vi "sum line into array.vi"(9 "insert location":i32, 10 "array to sum in":u32[](array[numeric]), 11 "array":u32[](array[numeric])) -> (3 "array out":u32[](array[numeric]))   [LabVIEW 2010]
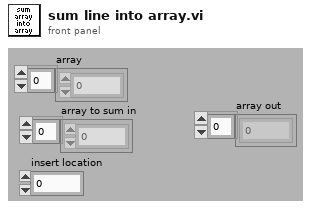
[diagram p1: front panel]
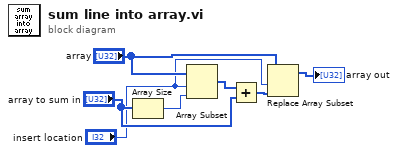
[diagram p0: block diagram]
diagram:
  n1 = Array Size(array="array to sum in") -> (size(s)=w7:i32)
  n2 = Array Subset(array="array", index="insert location", length=w7) -> (w6:u32[])
  n3 = Add(x=w6, y="array to sum in") -> (x+y=w2:u32[])
  n4 = Replace Array Subset(array="array", new element=w2, index="insert location") -> (→"array out":u32[])
